vi "Photodetector DAQ with triggering.vi"() -> ()   [LabVIEW 2018]
uses:
  <vilib>/DAQmx/read.llb/DAQmx Read (Analog 1D Wfm NChan NSamp).vi
  <vilib>/Analysis/8numeric.llb/1D Numeric Integration.vi
  <vilib>/DAQmx/create/channels.llb/DAQmx Create Channel (AI-Voltage-Basic).vi
  <vilib>/DAQmx/configure/timing.llb/DAQmx Timing (Sample Clock).vi
  <vilib>/DAQmx/configure/trigger.llb/DAQmx Start Trigger (Digital Edge).vi
  <vilib>/DAQmx/miscellaneous.llb/DAQmx Fill In Error Info.vi
  <vilib>/Waveform/WDTOps.llb/WDT Index Channel by Name DBL.vi
  <vilib>/Analysis/NI_AALPro.lvlib
panel:
  out "Minimum of absorption signal":dbl[](graph)
  out "Integral of PMT signal":dbl[](graph)
  out "Waveform Graph":waveform(dbl)[](graph)
  in  "Save data?":bool
  in  "file path (dialog if empty)":path=path "C:/Users/Oskari/Google Drive/CeNTREX Oskari/TlF beam profiling/Data acquisition software/LabView/test.csv"
  out "Error message message":string=" INSTRUCTIONS:\r\rNormal Use:  When using subVIs that incorporate the error in/error out (or error I/O) structure, place this handler where you want to inform the user of an error, typically at the end of the I/O data path, as the last action of the program.  If the error in error? is ERROR, the handler creates a message describing the error and its source.  If the type of dialog = 1 (default), the message is displayed to the user, who can only acknowedge it.  If the type = 2, the user can acknowledge the message or abort execution; aborting a program with active I/O is not recommended.  If the type = 0, no message is displayed; this is used to process the error programmatically, and the error out cluster elements are wired to individual terminals for that reason.  \r\rOther Use:\n\r\nlocal testing.  To test the error code of a subVI or function that does not have the error I/O structure, you can wire its error code and a source string to the local error code and error source inputs.  If error in error? indicates no error and error code is not equal to 0, the local code and source are substituted for the error in values, and error? is set TRUE (ERROR)."
  in  "stop":bool
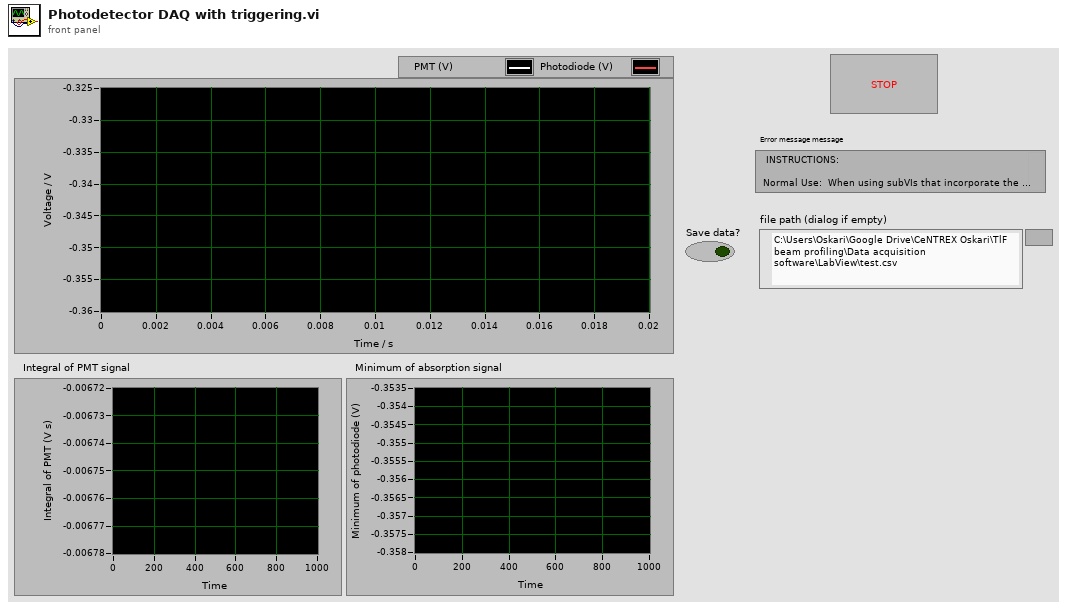
[diagram p1: front panel]
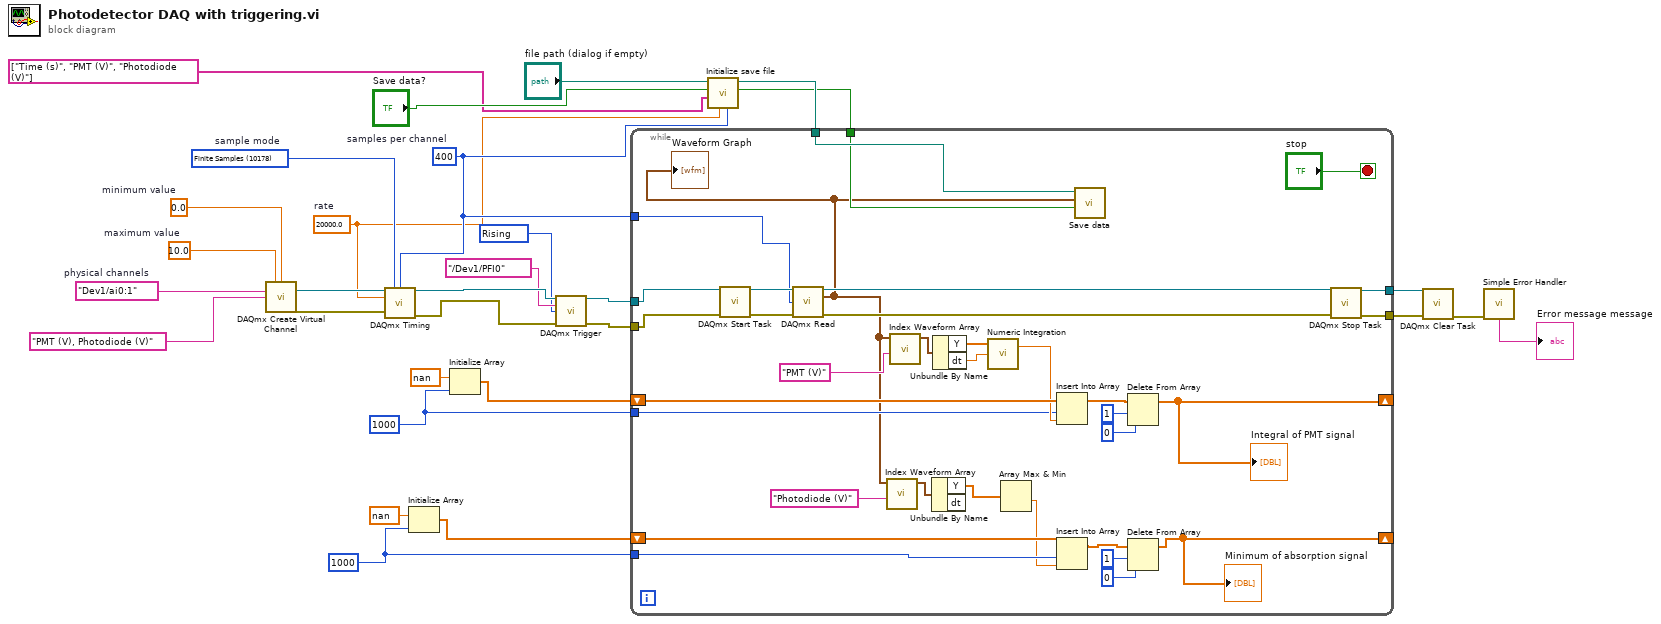
[diagram p0: block diagram]
diagram:
  w5 = 10280 items=["Rising"=10280, "Falling"=10171] ("edge")
  w14 = 1000 ("dimension size")
  w17 = 1000 ("dimension size")
  w9 = 400  # samples per channel
  w25 = 10178 items=["Finite Samples"=10178, "Continuous Samples"=10123, "Hardware Timed Single Point"=12522]  # sample mode
  w8 = 20000.0  # rate
  w28 = 0.0  # minimum value
  w29 = 10.0  # maximum value
  w30 = tag "Dev1/ai0:1"  # physical channels
  n1 = call-poly <vilib>:"DAQmx Create Virtual Channel.vi"("maximum value"=w29, "minimum value"=w28, "physical channels"=w30, "name to assign"="PMT (V), Photodiode (V)") -> ("task out"=w27:refnum<k21>, "error out"=w26:errorcluster)  [unwired: 10 in]
  n2 = call-poly <vilib>:"DAQmx Timing.vi"("task/channels in"=w27, "sample mode"=w25, "samples per channel"=w9, "rate"=w8, "error in"=w26) -> ("task out"=w7:refnum<k21>, "error out"=w4:errorcluster)  [unwired: 9 in]
  n3 = Initialize Array(nan ("element"), w14) -> (w15:dbl[])
  n4 = Initialize Array(nan ("element"), w17) -> (w18:dbl[])
  n5 = call-poly <vilib>:"DAQmx Trigger.vi"("task/channels in"=w7, "source"=tag "/Dev1/PFI0", "edge"=w5, "error in"=w4) -> ("task out"=w3:refnum<k21>, "error out"=w2:errorcluster)  [unwired: 10 in]
  n6 = call "Initialize save file.vi"("Number of samples per channel"=w9, "Sampling rate"=w8, "Headers"=string[] ["Time (s)", "PMT (V)", "Photodiode (V)"], "Save data? in"="Save data?", "Save data path in"="file path (dialog if empty)") -> ("Save data? out"=w11:bool, "Save data path out"=w12:path)  [unwired: 4 in, 1 out]
  n7 = while {
    tunnel: [w62] -> w24
    tunnel: [w61] -> w23
    tunnel: w12 -> [w59]
    tunnel: w11 -> [w57]
    tunnel: w9 -> [w33]
    tunnel: w17 -> [w49]
    shift-right: [w35] -> _
    shift-left: w18 -> [w51]
    tunnel: w14 -> [w40]
    shift-right: [w34] -> _
    shift-left: w15 -> [w41]
    tunnel: w3 -> [w32]
    tunnel: w2 -> [w31]
    stop <- "stop" stop-if-true
    n8 = call <vilib>:"DAQmx Start Task.vi"("task/channels in"=w32, "error in"=w31) -> ("task out"=w64:refnum<k21>, "error out"=w63:errorcluster)  [unwired: 12 in]
    n9 = call-poly <vilib>:"DAQmx Read.vi"("task/channels in"=w64, "number of samples per channel"=w33, "error in"=w63) -> ("task out"=w60:refnum<k21>, "data"=w45:waveform(dbl)[], "error out"=w58:errorcluster)  [unwired: 10 in]
    "Waveform Graph" <- w45
    n10 = call-poly <vilib>:"Index Waveform Array.vi"("channel name"="Photodiode (V)" ("index"), "waveform array"=w45) -> ("waveform"=w43:waveform(dbl))  [unwired: 8 in, 1 out]
    n11 = call-poly <vilib>:"Index Waveform Array.vi"("channel name"="PMT (V)" ("index"), "waveform array"=w45) -> ("waveform"=w54:waveform(dbl))  [unwired: 8 in, 1 out]
    n12 = Unbundle By Name(w43) -> ("Y"=w42:dbl[])  [unwired: 1 out]
    n13 = Unbundle By Name(w54) -> ("Y"=w53:dbl[], "dt"=w52:dbl)
    n14 = call-poly <vilib>:"Numeric Integration.vi"("dt"=w52, "Input Array"=w53) -> ("result"=w50:dbl)  [unwired: 1 in, 1 out]
    n15 = Array Max & Min(array=w42) -> (min value=w39:dbl)  [unwired: 3 out]
    n16 = Insert Into Array(array=w51, index=w49, new element=w50) -> (w48:dbl[])
    n17 = Insert Into Array(array=w41, index=w40, new element=w39) -> (w36:dbl[])
    n18 = call "Save data.vi"("Save data?"=w57, "data"=w45, "file path (dialog if empty)"=w59) -> ()  [unwired: 8 in, 1 out]
    n19 = Delete From Array(array=w48, length=1, index=0) -> (array with subset deleted=w35:dbl[])  [unwired: 1 out]
    "Integral of PMT signal" <- w35
    n20 = Delete From Array(array=w36, length=1, index=0) -> (array with subset deleted=w34:dbl[])  [unwired: 1 out]
    "Minimum of absorption signal" <- w34
    n21 = call <vilib>:"DAQmx Stop Task.vi"("task/channels in"=w60, "error in"=w58) -> ("task out"=w62:refnum<k21>, "error out"=w61:errorcluster)  [unwired: 12 in]
  }
  n22 = call <vilib>:"DAQmx Clear Task.vi"("task in"=w24, "error in"=w23) -> ("error out"=w22:errorcluster)  [unwired: 13 in]
  n23 = call <vilib>:"Simple Error Handler.vi"("error in (no error)"=w22) -> ("message"=→"Error message message":string)  [unwired: 4 in, 4 out]
